vi "FPGA_DAC_buses.vi"() -> ()   [LabVIEW 2013]
uses:
  <vilib>/rvi/Emulation/niFpgaSctlEmulationGetInTimedLoop.vi
  <vilib>/rvi/Emulation/niFpgaEmulationReportErrorSimple.vi
  <vilib>/rvi/Emulation/niFpgaGetClockAttributes.vi
  <vilib>/rvi/FIFO/Fifo_Resource/nirvififoEmulationReadFpgaImpl.vi
  <vilib>/rvi/DataTransferAndStorage/Container/Common/niFpgaContainerGetUniqueNameForEmu.vi
  <vilib>/rvi/Emulation/niFpgaProcessEmulError.vi
  <vilib>/rvi/Memory/Memory_Emulation/nirvimemoryEmulation.vi
  <vilib>/rvi/Memory/Memory_Emulation/nirvimemoryFastEmulation.vi
  <vilib>/rvi/Memory/Memory_Emulation/niFpgaMemoryEmulationCacheClearOnFirstRun.vi
  <vilib>/rvi/Memory/Memory_Emulation/nirvimemoryEmulationManagerCache_MakeExclusive.vi
  <vilib>/rvi/Memory/Memory_Emulation/niFpgaMemoryEmulationValidateCache.vi
  <vilib>/rvi/Memory/Memory_Emulation/nirvimemoryEmulationManagerCache_ReleaseExclusive.vi
  <vilib>/rvi/Memory/Memory_Emulation/nirvimemoryEmulationManagerCache_InsertValue.vi
  <vilib>/Utility/error.llb/Clear Errors.vi
  <vilib>/rvi/Memory/Memory_Emulation/nirvimemoryEmulationManagerCache_SetValue.vi
  <vilib>/rvi/Emulation/niFpgaSctlEmulationResourceMgr.vi
  <vilib>/rvi/Emulation/niFpgaCriticalErrorInLSC.vi
  <vilib>/rvi/Memory/Memory_Emulation/nirvimemoryEmulationManagerCache_GetValue.vi
  <vilib>/rvi/FIFO/Fifo_Resource/nirvififoEmulationWriteFpgaImpl.vi
  <vilib>/rvi/DataTransferAndStorage/Container/XNode/niFpgaContainer.xnode
  <vilib>/rvi/FIFO/Fifo_Resource/nirvififoEmulationRead.vi
  <vilib>/rvi/FIFO/Fifo_Resource/nirvififoEmulationWrite.vi
panel:
  in  "start movement":bool
  in  "buses to use":bool[](array[boolean])=[FALSE, FALSE, FALSE, FALSE, FALSE, FALSE, FALSE, FALSE]
  in  "wait(mSec)":u8
  in  "stop moving bus":bool
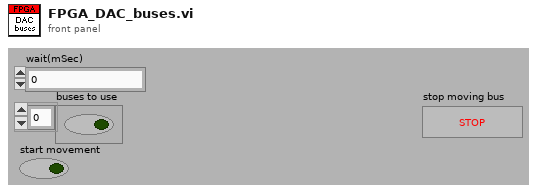
[diagram p1: front panel]
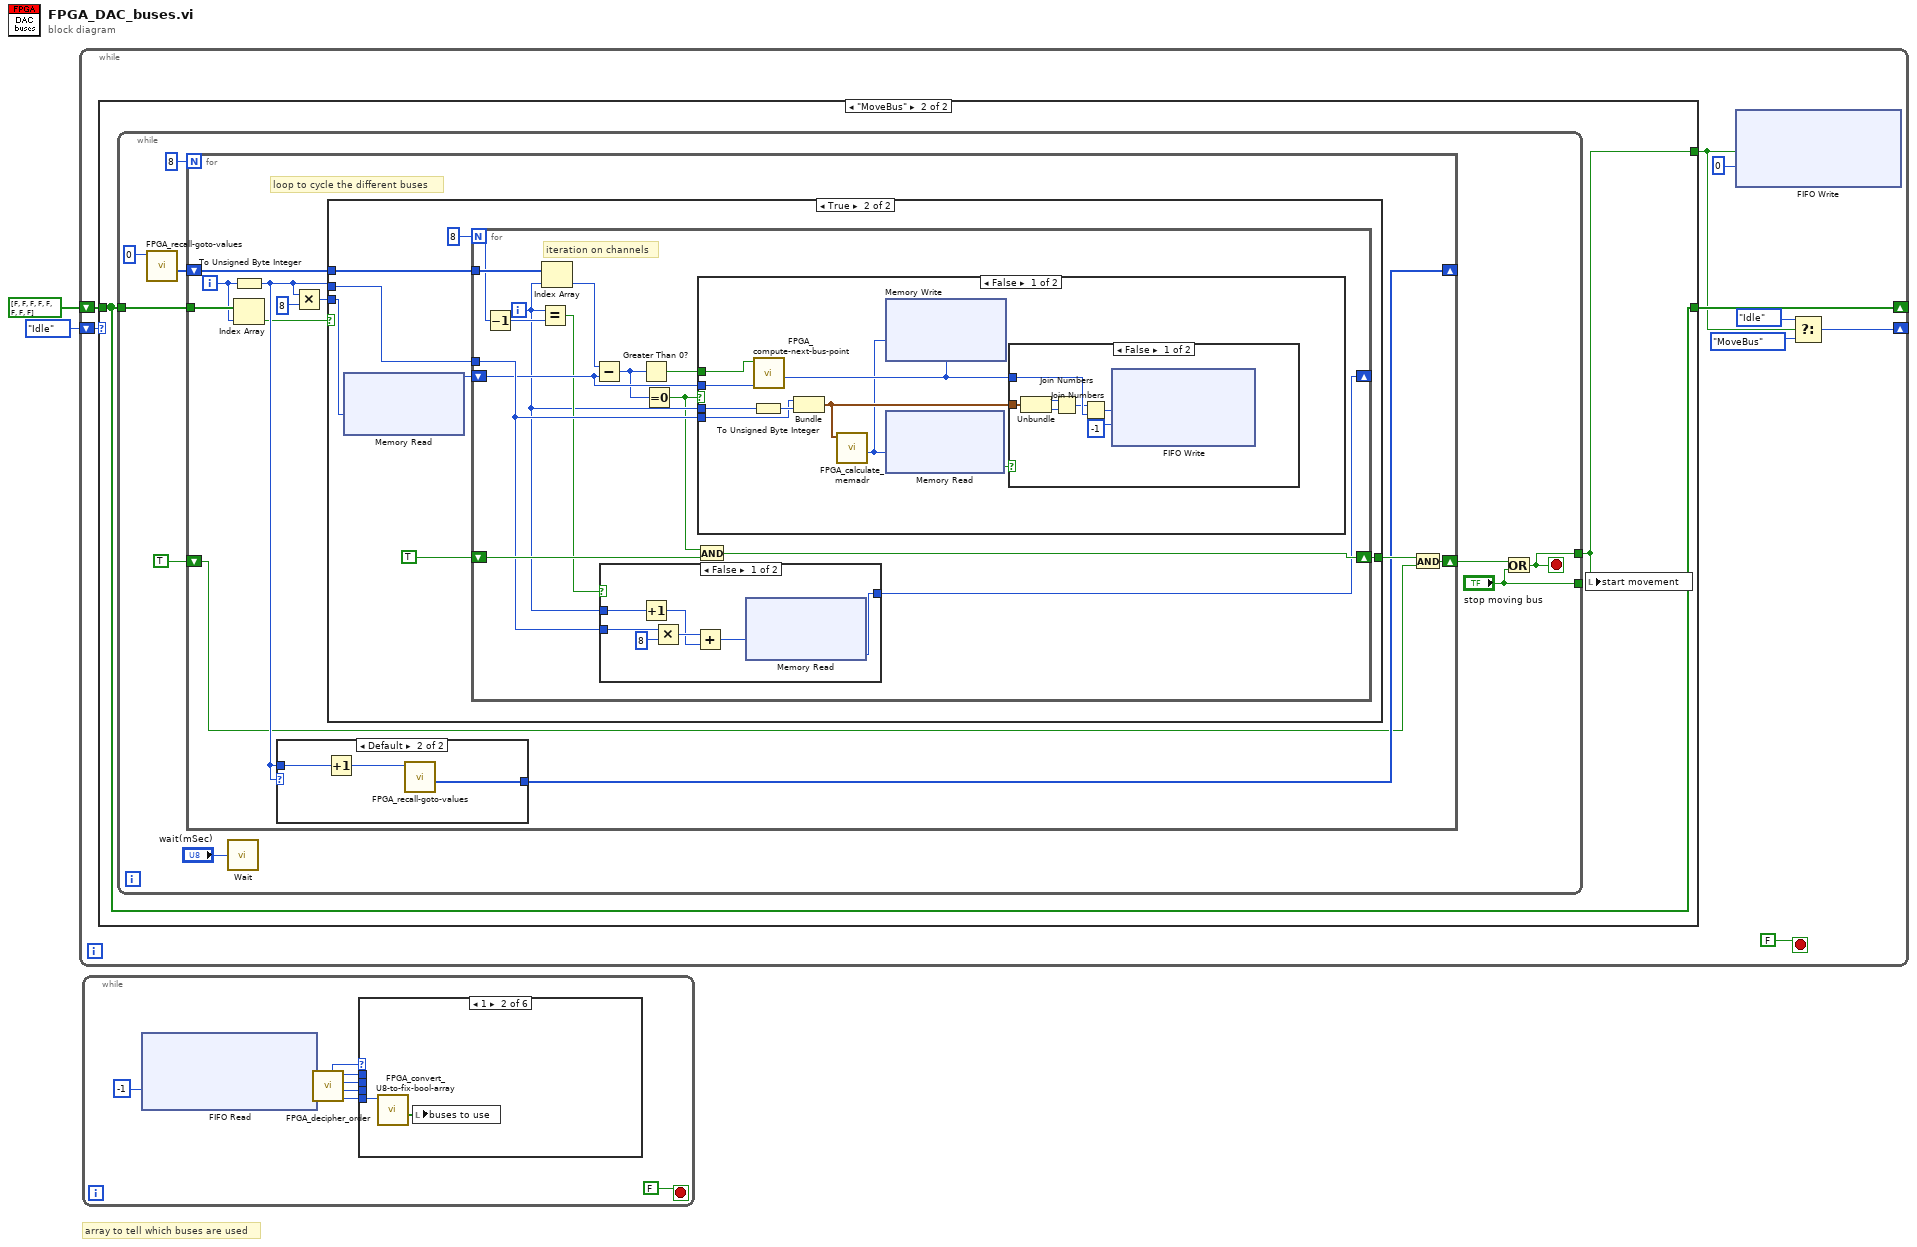
[diagram p0: block diagram]
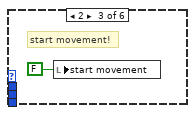
[diagram p3: hidden frame]
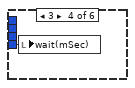
[diagram p4: hidden frame]
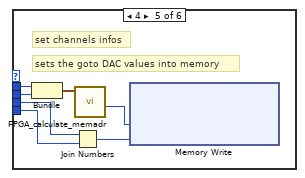
[diagram p5: hidden frame]
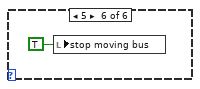
[diagram p6: hidden frame]
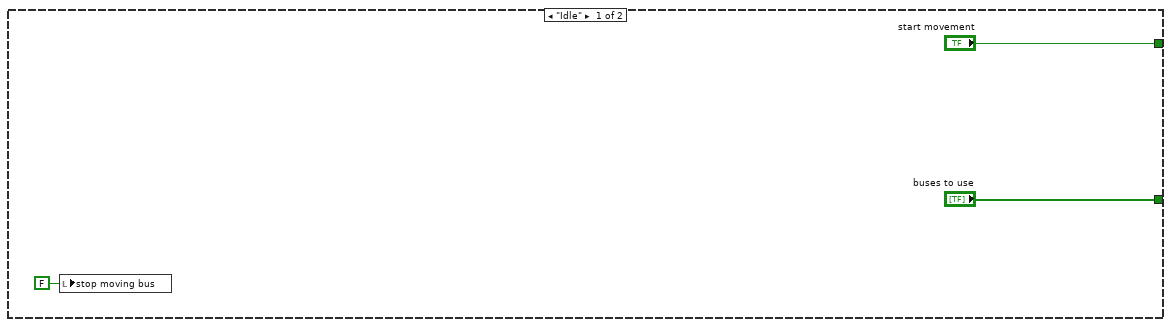
[diagram p7: hidden frame]
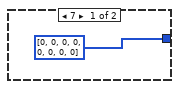
[diagram p8: hidden frame]
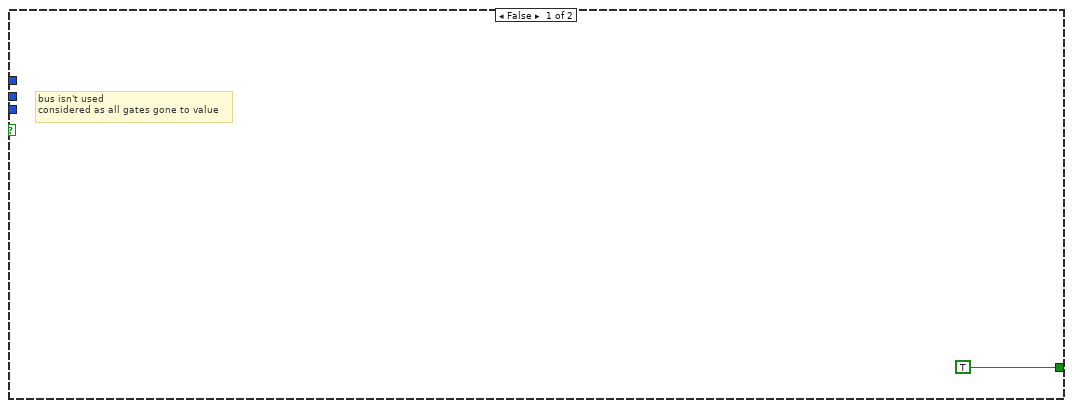
[diagram p9: hidden frame]
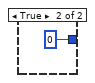
[diagram p10: hidden frame]
diagram:
  # "array to tell which buses are used"
  n1 = while {
    shift-right: [w8] -> _
    shift-left: enum16{"Idle", "MoveBus"}."Idle" -> [w11]
    shift-right: [w5] -> _
    shift-left: bool[] [FALSE, FALSE, FALSE, FALSE, FALSE, FALSE, FALSE, FALSE] -> [w6]
    stop <- FALSE stop-if-true
    n2 = case shown="\"MoveBus\"" w11 {
      tunnel: ["start movement" w15] -> w4
      tunnel: w6 -> [_ w16]
      tunnel: ["buses to use" w16] -> w5
      frame "Idle" {
        n3 = local write "stop moving bus"(FALSE ("stop moving bus")) -> ()
      }
      frame "MoveBus" {
        n4 = while {
          tunnel: ["stop moving bus"] -> _
          tunnel: [w24] -> w15
          tunnel: w16 -> [w20]
          stop <- w24 stop-if-true
          n5 = call "FPGA_recall-goto-values.vi"("panel"=u8 0) -> ("bus' goto values"=w18:u16[])  [unwired: 10 out]
          n6 = for {
            N: 8 -> [_]
            shift-right: [w35] -> w22
            shift-left: TRUE -> [w26]
            tunnel: w20 -> [w34]
            shift-right: [w30] -> _
            shift-left: w18 -> [w31]
            i -> [w27]
            # "loop to cycle the different buses"
            n7 = To Unsigned Byte Integer(number=w27) -> (unsigned 8bit integer=w29:u8)
            n8 = Index Array(array=w34, index=w27) -> (element=w28:bool)
            n9 = case shown="Default" w29 {
              tunnel: w29 -> [_ w40]
              tunnel: [u16[] [0, 0, 0, 0, 0, 0, 0, 0] ("bus' goto values") w38] -> w30
              frame 7 {
              }
              frame Default {
                n10 = Increment(x=w40) -> (x+1=w39:u8)
                n11 = call "FPGA_recall-goto-values.vi"("panel"=w39) -> ("bus' goto values"=w38:u16[])  [unwired: 10 out]
              }
            }
            n12 = Multiply(x=w29, y=u8 8) -> (x*y=w32:u8)
            n13 = case shown="True" w28 {
              tunnel: w31 -> [_ w45]
              tunnel: [TRUE w44] -> w36
              tunnel: w29 -> [_ w43]
              tunnel: w32 -> [_ w42]
              frame False {
                # "bus isn't used\nconsidered as all gates gone to value"
              }
              frame True {
                n14 = xnode ("Memory Read")("Address"=w42) -> ("Data"=w46:u16)  [unwired: 1 in, 1 out]
                n15 = for {
                  N: 8 -> [w56]
                  tunnel: w43 -> [w59]
                  tunnel: w45 -> [w62]
                  shift-right: [w60] -> w44
                  shift-left: TRUE -> [w61]
                  shift-right: [w57] -> _
                  shift-left: w46 -> [w58]
                  i -> [w52]
                  # "iteration on channels"
                  n16 = Decrement(x=w56) -> (x-1=w54:i32)
                  n17 = Equal?(x=w52, y=w54) -> (x = y?=w55:bool)
                  n18 = Index Array(array=w62, index=w52) -> (element=w53:u16)
                  n19 = Subtract(x=w53, y=w58) -> (x-y=w50:i32)
                  n20 = case shown="False" w55 {
                    tunnel: w59 -> [w69 _]
                    tunnel: w52 -> [w67 _]
                    tunnel: [w64 u16 0 ("Data")] -> w57
                    frame False {
                      n21 = Increment(x=w67) -> (x+1=w63:i32)
                      n22 = Multiply(x=w69, y=u8 8) -> (x*y=w68:u8)
                      n23 = Add(x=w68, y=w63) -> (x+y=w65:u8)
                      n24 = xnode ("Memory Read")("Address"=w65) -> ("Data"=w64:u16)  [unwired: 1 in, 1 out]
                    }
                    frame True {
                    }
                  }
                  n25 = Greater Than 0?(x=w50) -> (x > 0?=w49:bool)
                  n26 = Equal To 0?(x=w50) -> (x = 0?=w51:bool)
                  n27 = And(x=w51, y=w61) -> (x .and. y?=w60:bool)
                  n28 = case shown="False" w51 {
                    tunnel: w59 -> [w71 _]
                    tunnel: w52 -> [w72 _]
                    tunnel: w58 -> [w79 _]
                    tunnel: w49 -> [w75 _]
                    frame False {
                      n29 = To Unsigned Byte Integer(number=w72) -> (unsigned 8bit integer=w78:u8)
                      n30 = call "FPGA_compute-next-bus-point.vi"("channel actual"=w79, "increase value"=w75) -> ("next point"=w76:u16)  [unwired: 9 out]
                      n31 = Bundle(w71, w78) -> (w77:cluster{u8, u8})  [unwired: 1 out]
                      n32 = call "FPGA_calculate_memadr.vi"("Cluster"=w77) -> ("mem adr"=w73:u8)  [unwired: 10 out]
                      n33 = xnode ("Memory Write")("Address"=w73, "Data"=w76) -> ()  [unwired: 1 in, 1 out]
                      n34 = xnode ("Memory Read")("Address"=w73) -> ("Data"=w74:bool)  [unwired: 1 in, 1 out]
                      n35 = case shown="False" w74 {
                        tunnel: w77 -> [w85 _]
                        tunnel: w76 -> [w82 _]
                        frame False {
                          n36 = Unbundle(w85) -> (w83:u8, w84:u8)
                          n37 = Join Numbers(hi=w83, lo=w84) -> ((hi.lo)=w81:u16)
                          n38 = Join Numbers(hi=w81, lo=w82) -> ((hi.lo)=w80:u32)
                          n39 = xnode ("FIFO Write")("Element"=w80, "Timeout"=-1) -> ()  [unwired: 1 in, 2 out]
                        }
                        frame True {
                        }
                      }
                    }
                    frame True {
                    }
                  }
                }
              }
            }
            n40 = And(x=w36, y=w26) -> (x .and. y?=w35:bool)
          }
          n41 = call "Wait"("Count(mSec)"="wait(mSec)") -> ()  [unwired: 1 out]
          n42 = Or(x=w22, y="stop moving bus") -> (x .or. y?=w24:bool)
        }
        n43 = local write "start movement"(w15) -> ()
      }
    }
    n44 = xnode ("FIFO Write")("Element"=w4, "Timeout"=0) -> ()  [unwired: 1 in, 2 out]
    n45 = Select(t=enum16{"Idle", "MoveBus"}."Idle", s=w4, f=enum16{"Idle", "MoveBus"}."MoveBus") -> (s? t:f=w8:enum16{"Idle", "MoveBus"})
  }
  n46 = while {
    stop <- FALSE stop-if-true
    n47 = xnode ("FIFO Read")("Timeout"=-1) -> ("Element"=w94:u64)  [unwired: 1 in, 2 out]
    n48 = call "FPGA_decipher_order.vi"("order in"=w94) -> ("data 1"=w90:u8, "data 2"=w87:u8, "data 3"=w89:u8, "data 4"=w88:u8, "order out"=w91:u8)  [unwired: 6 out]
    n49 = case shown="1" w91 {
      tunnel: w90 -> [_ w96 _ w98 w100 _]
      tunnel: w89 -> [_ _ _ _ w103 _]
      tunnel: w88 -> [_ _ _ _ w102 _]
      tunnel: w87 -> [_ _ _ _ w99 _]
      frame 0, Default {
      }
      frame 1 {
        n50 = call "FPGA_convert_U8-to-fix-bool-array.vi"("U8"=w96) -> ("bool array"=w95:bool[])  [unwired: 10 out]
        n51 = local write "buses to use"(w95) -> ()
      }
      frame 2 {
        # "start movement!"
        n52 = local write "start movement"(FALSE ("start movement")) -> ()
      }
      frame 3 {
        n53 = local write "wait(mSec)"(w98) -> ()
      }
      frame 4 {
        # "sets the goto DAC values into memory"
        # "set channels infos"
        n54 = Bundle("data 4"=w102, "data 3"=w103) -> (w105:cluster{"data 4":u8, "data 3":u8})  [unwired: 1 out]
        n55 = Join Numbers(hi=w99, lo=w100) -> ((hi.lo)=w101:u16)
        n56 = call "FPGA_calculate_memadr.vi"("Cluster"=w105) -> ("mem adr"=w104:u8)  [unwired: 10 out]
        n57 = xnode ("Memory Write")("Address"=w104, "Data"=w101) -> ()  [unwired: 1 in, 1 out]
      }
      frame 5 {
        n58 = local write "stop moving bus"(TRUE ("stop moving bus")) -> ()
      }
    }
  }
